vi "Query TrigLevel.vi"(8 "error in (no error)":errorcluster, 11 "CS++MCS in":refnum<class "CS++MCS.lvclass">) -> (0 "error out":errorcluster, 2 "Trigger Level":dbl[unit], 3 "CS++MCS out":refnum<class "CS++MCS.lvclass">)   [LabVIEW 2016, in "CS++MCS.lvlib" / "CS++MCS.lvclass"]
doc: "This VI reads out the Trigger Level from the device."
uses:
  CS++MCS.lvclass
  CSPP_Core/Classes/CS++ProcessVariables/ProcessVariable/PV.lvclass
  PV-Enum.ctl
  CSPP_Core/Classes/CS++ProcessVariables/ProcessVariable/PV.lvclass/PV.ctl
  CS++MCS.lvclass/CS++MCS.ctl
  CSPP_Core/Classes/CS++ProcessVariables/ProcessVariable/Write Data.vi
  CSPP_Core/Classes/CS++ProcessVariables/ProcessVariable/Write Timestamp.vi
  CSPP_Core/Classes/CS++ProcessVariables/ProcessVariable/Write Quality.vi
  CSPP_Core/Classes/CS++ProcessVariables/ProcessVariable/Write status.vi
  CSPP_Core/Classes/CS++ProcessVariables/PVConnection/PVConnection.lvclass
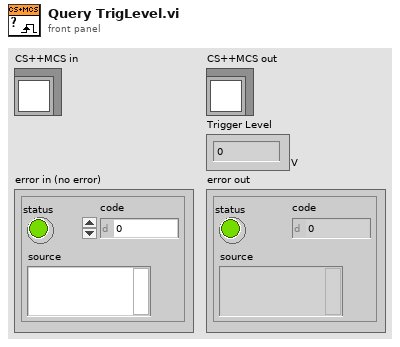
[diagram p1: front panel]
types:
  T1 = typedef "CS++MCS.lvlib/CS++MCS.lvclass/PV-Enum.ctl" = enum16{"Counts/I32", "TotalCounts/I32", "Status/I8", "BinWidth/Dbl", "NofBins/I32", "NofRecords /I32", "DiscLvl/Dbl", "TrigLvl/Dbl", "DiscSlope/U16", "TrigSlope/U16", "ActWaveform/AWfm|0:1"}
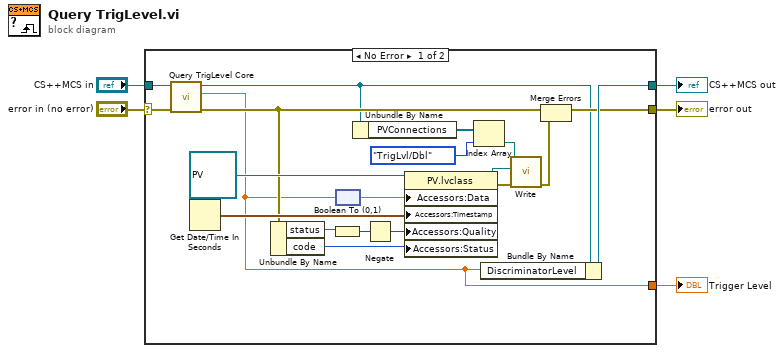
[diagram p0: block diagram]
diagram:
  n1 = case shown="No Error" "error in (no error)" {
    selector: "error in (no error)" -> [w10 w27]
    tunnel: [w11 w27] -> w4
    tunnel: [w12 w26] -> w2
    tunnel: "CS++MCS in" -> [w8 w26]
    tunnel: [w6 _] -> w1
    frame No Error {
      n2 = call-dynamic "Query TrigLevel Core.vi"("error in (no error)"=w10, "CS++MCS in"=w8) -> ("error out"=w9:errorcluster, "Trigger Level"=w6:dbl[unit], "CS++MCS out"=w7:refnum<class "CS++MCS.lvclass">)  [unwired: 7 in]
      n3 = Get Date/Time In Seconds() -> (seconds since 1Jan1904=w17:timestamp)
      n4 = Unbundle By Name(w9) -> ("status"=w21:bool, "code"=w23:i32)
      n5 = Boolean To (0,1)(Boolean=w21) -> (0, 1=w22:i16)
      n6 = node(w6) -> (w14:dbl)
      n7 = Unbundle By Name(w7) -> ("PVConnections"=w25:refnum<class "PVConnection.lvclass">[])
      n8 = Negate(x=w22) -> (-x=w24:i16)
      n9 = property class="PV.lvclass"(reference=refnum<class "PV.lvclass"> refnum ("PV"), "Accessors:Data"=w14, "Accessors:Timestamp"=w17, "Accessors:Quality"=w24, "Accessors:Status"=w23) -> (reference out=w20:refnum<class "PV.lvclass">, error out=w19:errorcluster)  [unwired: 1 in]
      n10 = Index Array(array=w25, index=PV-Enum."TrigLvl/Dbl" ("PV-Enum")) -> (element=w16:refnum<class "PVConnection.lvclass">)
      n11 = Bundle By Name(cluster=w7, "DiscriminatorLevel"=w6) -> (w12:refnum<class "CS++MCS.lvclass">)
      n12 = call "Write.vi"("error in (no error)"=w19, "PV"=w20, "PVConnection in"=w16) -> ("error out"=w15:errorcluster)  [unwired: 7 in, 1 out]
      n13 = Merge Errors(w9, w15) -> (w11:errorcluster)
    }
    frame Error {
    }
  }
  "error out" <- w4
  "CS++MCS out" <- w2
  "Trigger Level" <- w1
